vi "ERR Error Global.vi"() -> ()   [LabVIEW 2011]
doc: "This vi was created by David Gianetto, contact me with any problems, questions, etc."
panel:
  in  "Log Queue":refnum<queue>
  out "Error Item Matrix":string[][](array[string])
  out "Error Description":string[](array[string])
  out "Error Level Array":i32[](array[numeric])
  out "Error Code Array":i32[](array[numeric])
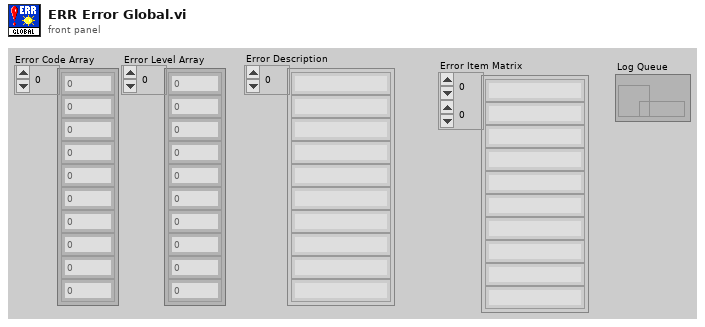
[diagram p1: front panel]
diagram:
